vi "Update Nested Tag.vi"(8 "error in (no error)":errorcluster, 9 "Data":variant, 10 "Path":cluster{"Tag ID / Name":variant, "Index":i32}[](array[cluster]), 11 "Raw Message in":refnum<class "Raw Message.lvclass">) -> (0 "error out":errorcluster, 3 "Raw Message out":refnum<class "Raw Message.lvclass">)   [LabVIEW 2020, in "Protobuf RAW.lvlib" / "Raw Message.lvclass"]
uses:
  Raw Message.lvclass
  E:/Labview/LV 2020/Libs/LV Protobuf Raw/Source/Tag/Basic Type.lvclass
  Raw Message.lvclass/Raw Message.ctl
  <vilib>/Utility/Data Type/Get Type Information.vi
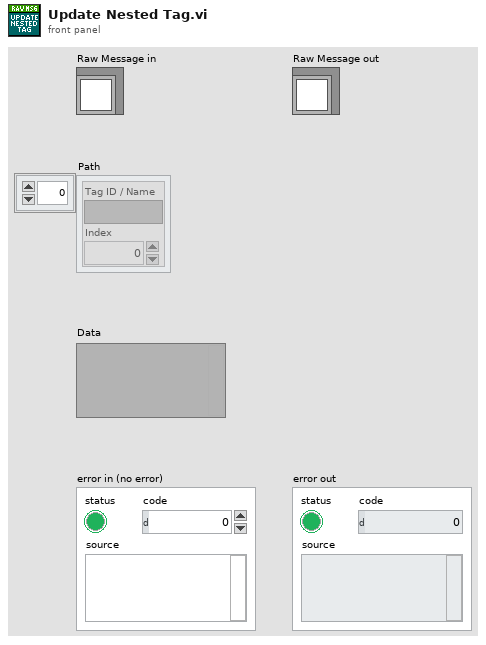
[diagram p1: front panel]
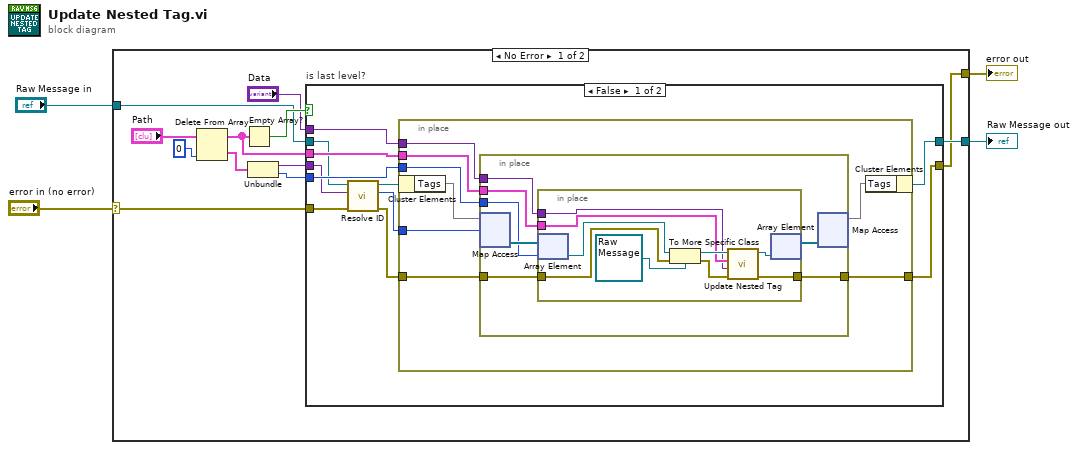
[diagram p0: block diagram]
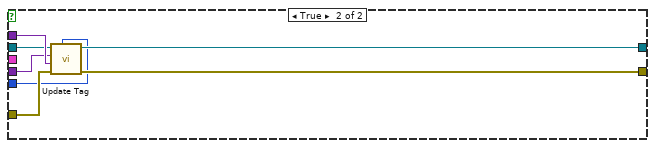
[diagram p2: hidden frame]
diagram:
  n1 = case shown="No Error" "error in (no error)" {
    selector: "error in (no error)" -> [w8 w59]
    tunnel: [w5 w59] -> w4
    tunnel: [w16 _] -> w1
    tunnel: "Raw Message in" -> [w6 _]
    frame No Error {
      n2 = Delete From Array(array="Path", index=0) -> (deleted portion=w13:cluster{"Tag ID / Name":variant, "Index":i32}, array with subset deleted=w11:cluster{"Tag ID / Name":variant, "Index":i32}[])  [unwired: 1 in]
      n3 = Empty Array?(array=w11) -> (empty?=w10:bool)
      n4 = Unbundle(w13) -> ("Tag ID / Name"=w7:variant, "Index"=w12:i32)
      n5 = case "is last level?" shown="False" w10 {
        tunnel: [w27 w57] -> w16
        tunnel: w12 -> [w26 w52]
        tunnel: w11 -> [w25 _]
        tunnel: [w24 w58] -> w5
        tunnel: "Data" -> [w23 w56]
        tunnel: w8 -> [w22 w53]
        tunnel: w7 -> [w21 w55]
        tunnel: w6 -> [w20 w54]
        frame False {
          n6 = call "Resolve ID.vi"("error in (no error)"=w22, "Tag ID / Name"=w21, "Raw Message in"=w20) -> ("error out"=w19:errorcluster, "Tag ID"=w18:u32, "Raw Message out"=w17:refnum<class "Raw Message.lvclass">)  [unwired: 6 in]
          n7 = in-place {
            in-place-border: w18 -> [w33]
            in-place-border: w26 -> [w32]
            in-place-border: w19 -> [w31]
            in-place-border: w25 -> [w30]
            in-place-border: [w29] -> w24
            in-place-border: w23 -> [w28]
            n8 = in-place-cluster #1(w17) -> ("Tags"=w35:map{u32, refnum<class "Basic Type.lvclass">[]})
            n9 = in-place {
              in-place-border: w32 -> [w40]
              in-place-border: w31 -> [w39]
              in-place-border: w30 -> [w38]
              in-place-border: [w37] -> w29
              in-place-border: w28 -> [w36]
              n10 = in-place-map #2(w35, w33) -> (w42:refnum<class "Basic Type.lvclass">[])  [unwired: 1 in, 1 out]
              n11 = in-place {
                in-place-border: w39 -> [w47]
                in-place-border: w38 -> [w46]
                in-place-border: [w44] -> w37
                in-place-border: w36 -> [w43]
                n12 = in-place-array #3(w42, w40) -> (w51:refnum<class "Basic Type.lvclass">)
                n13 = To More Specific Class(target class=refnum<class "Raw Message.lvclass"> refnum ("Raw Message out"), reference=w51, error in=w47) -> (specific class reference=w50:refnum<class "Raw Message.lvclass">, error out=w49:errorcluster)
                n14 = call "Update Nested Tag.vi"("error in (no error)"=w49, "Data"=w43, "Path"=w46, "Raw Message in"=w50) -> ("error out"=w44:errorcluster, "Raw Message out"=w45:refnum<class "Raw Message.lvclass">)  [unwired: 6 in]
                n15 = in-place-array #3(w45) -> (w41:refnum<class "Basic Type.lvclass">[])  [unwired: 1 out]
              }
              n16 = in-place-map #2(w41) -> (w34:map{u32, refnum<class "Basic Type.lvclass">[]})  [unwired: 1 in, 2 out]
            }
            n17 = in-place-cluster #1("Tags"=w34) -> (w27:refnum<class "Raw Message.lvclass">)
          }
        }
        frame True {
          n18 = call "Update Tag.vi"("Index"=w52, "error in (no error)"=w53, "Variant"=w56, "Tag ID / Name"=w55, "Raw Message in"=w54) -> ("error out"=w58:errorcluster, "Raw Message out"=w57:refnum<class "Raw Message.lvclass">)  [unwired: 4 in, 1 out]
        }
      }
    }
    frame Error {
    }
  }
  "error out" <- w4
  "Raw Message out" <- w1
